vi "View.vi"(0 "object in":refnum<class "TDMS.lvclass">, 2 "Requirements":T2, 5 "Error In":errorcluster) -> (14 "object out":refnum<class "TDMS.lvclass">, 16 "Message":T1, 19 "Error Out":errorcluster)   [LabVIEW 2024, in "TDMS.lvclass"]
doc: "Opens an TDMS file and runs Viewer classes Execute method"
uses:
  TDMS.lvclass
  Support/Type Def/Requirements.ctl
  Support/Type Def/File Type.ctl
  Support/Type Def/Message.ctl
  IDataMethod_interface/IDataMethod.lvclass
panel:
  # "Connector Pane"
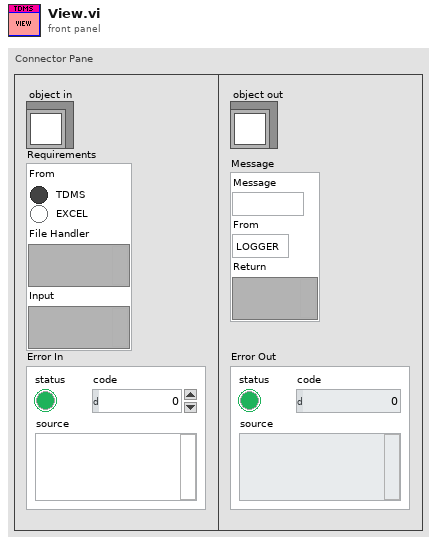
[diagram p1: front panel]
types:
  T1 = typedef "Message.ctl" = cluster{"Message":string, "From":enum16{"LOGGER", "VIEWER"}, "Return":variant}
  T2 = typedef "Requirements.ctl" = cluster{"From":T3, "File Handler":variant, "Input":variant}
  T3 = typedef "File Type.ctl" = enum32{"TDMS", "EXCEL"}
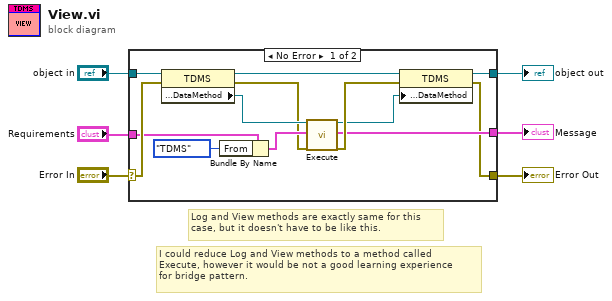
[diagram p0: block diagram]
diagram:
  # "I could reduce Log and View methods to a method called\nExecute, however it would be not a good learning experience\nfor bridge pattern."
  # "Log and View methods are exactly same for this\ncase, but it doesn't have to be like this."
  n1 = case shown="No Error" "Error In" {
    selector: "Error In" -> [w19 w21]
    tunnel: [w7 w21] -> w5
    tunnel: [w11 w20] -> w3
    tunnel: "object in" -> [w17 w20]
    tunnel: "Requirements" -> [w13 _]
    tunnel: [w8 _] -> w1
    frame No Error {
      n2 = property class="TDMS"(reference=w17, error in=w19) -> (reference out=w16:refnum<class "TDMS.lvclass">, error out=w12:errorcluster, "properties:DataMethod"=w14:refnum<class "IDataMethod.lvclass">)
      n3 = Bundle By Name(cluster=w13, "From"=enum16{"TDMS", "EXCEL"}."TDMS") -> (w15:T2)
      n4 = call-dynamic "Execute.vi"("object in"=w14, "Requirements"=w15, "Error In"=w12) -> ("object out"=w9:refnum<class "IDataMethod.lvclass">, "Message"=w8:T1, "Error Out"=w10:errorcluster)  [unwired: 14 in]
      n5 = property class="TDMS"(reference=w16, error in=w10, "properties:DataMethod"=w9) -> (reference out=w11:refnum<class "TDMS.lvclass">, error out=w7:errorcluster)
    }
    frame Error {
    }
  }
  "Error Out" <- w5
  "object out" <- w3
  "Message" <- w1
